vi "Swerve Global Variables.vi"() -> ()   [LabVIEW 2020]
doc: "Global variables in charge of the Swerve Drive subsystem."
panel:
  in  "Gyro Offset":dbl
  in  "Manual Output":dbl
  in  "Left Extention Motor":dbl
  in  "Right Extention Motor":dbl
  in  "Current Extention R":dbl
  in  "Current Extension L":dbl
  in  "L Rotate Motor":dbl
  in  "R Rotate Motor":dbl
  in  "Rotation Motor Threshold Right":dbl
  in  "Rotation Motor Threshold Left":dbl
  in  "Target Rotation Right":dbl
  in  "Target Rotation Left":dbl
  in  "Right Rotation Encoder":dbl
  in  "Left Rotation Encoder":dbl
  in  "Right Rotation Motor":dbl
  in  "Left Rotation Motor":dbl
  in  "Target Extension":dbl
  in  "Clamp":dbl
  in  "Manual Rotate In/Out":dbl
  in  "Manual Extend/Retract":dbl
  in  "Reset Gyro":bool
  in  "Use Field Oriented Controls":bool
  in  "Gyro Angle":dbl
  in  "Twist Axis":dbl
  in  "Y Axis":dbl
  in  "X Axis":dbl
  # "NOT SWERVE NEEDS \nTO BE MOVED"
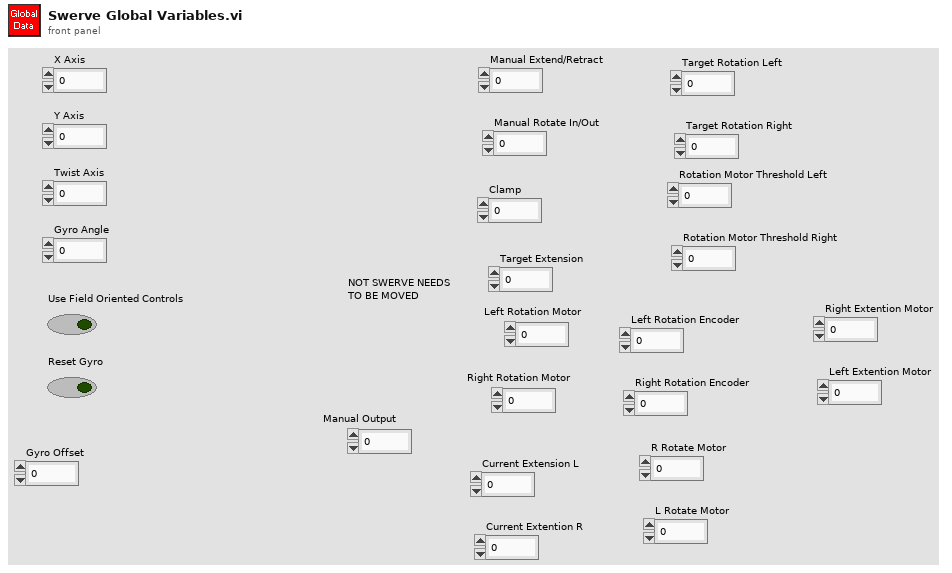
[diagram p1: front panel]
diagram:
